vi "Handle.vi"(8 "error in (no error)":errorcluster, 11 "Instrument in":refnum<class "Instrument.lvclass">) -> (0 "error out":errorcluster, 3 "Instrument out":refnum<class "Instrument.lvclass">)   [LabVIEW 2018, in "Instrument.lvclass"]
uses:
  Instrument.lvclass
  C:/Users/devstaff/sparc4/s4gui/Versao ZeroMQ REQ-REP/SPARC4_GUI -v1.0.0 - 20250122_ICS-JSON/Server/Server.lvclass
  Server/Server.lvclass/Server.ctl
  Instrument.lvclass/Instrument.ctl
  Device/Device.lvclass/Device.ctl
  Device/Optics/Opt_Selector/Opt_Selector.lvclass
  C:/Users/devstaff/sparc4/s4gui/Versao ZeroMQ REQ-REP/SPARC4_GUI -v1.0.0 - 20250122_ICS-JSON/Device/Device.lvclass
  Device/Optics/Opt_Continuous/Opt_Continuous.lvclass
  Server/Server.lvclass
  Comm/Stream/Stream.lvclass
  Device/Device.lvclass
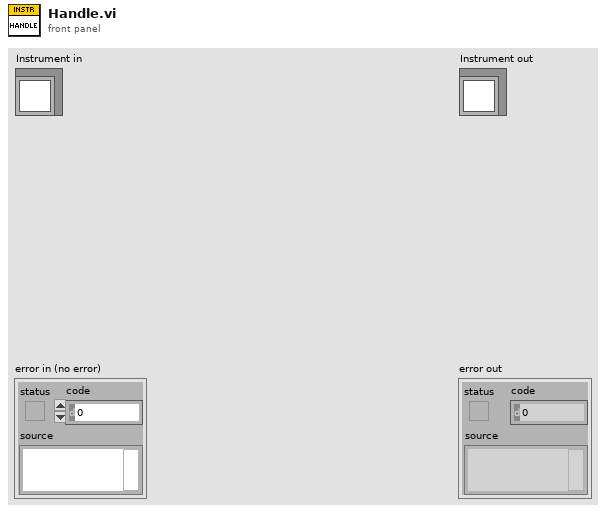
[diagram p1: front panel]
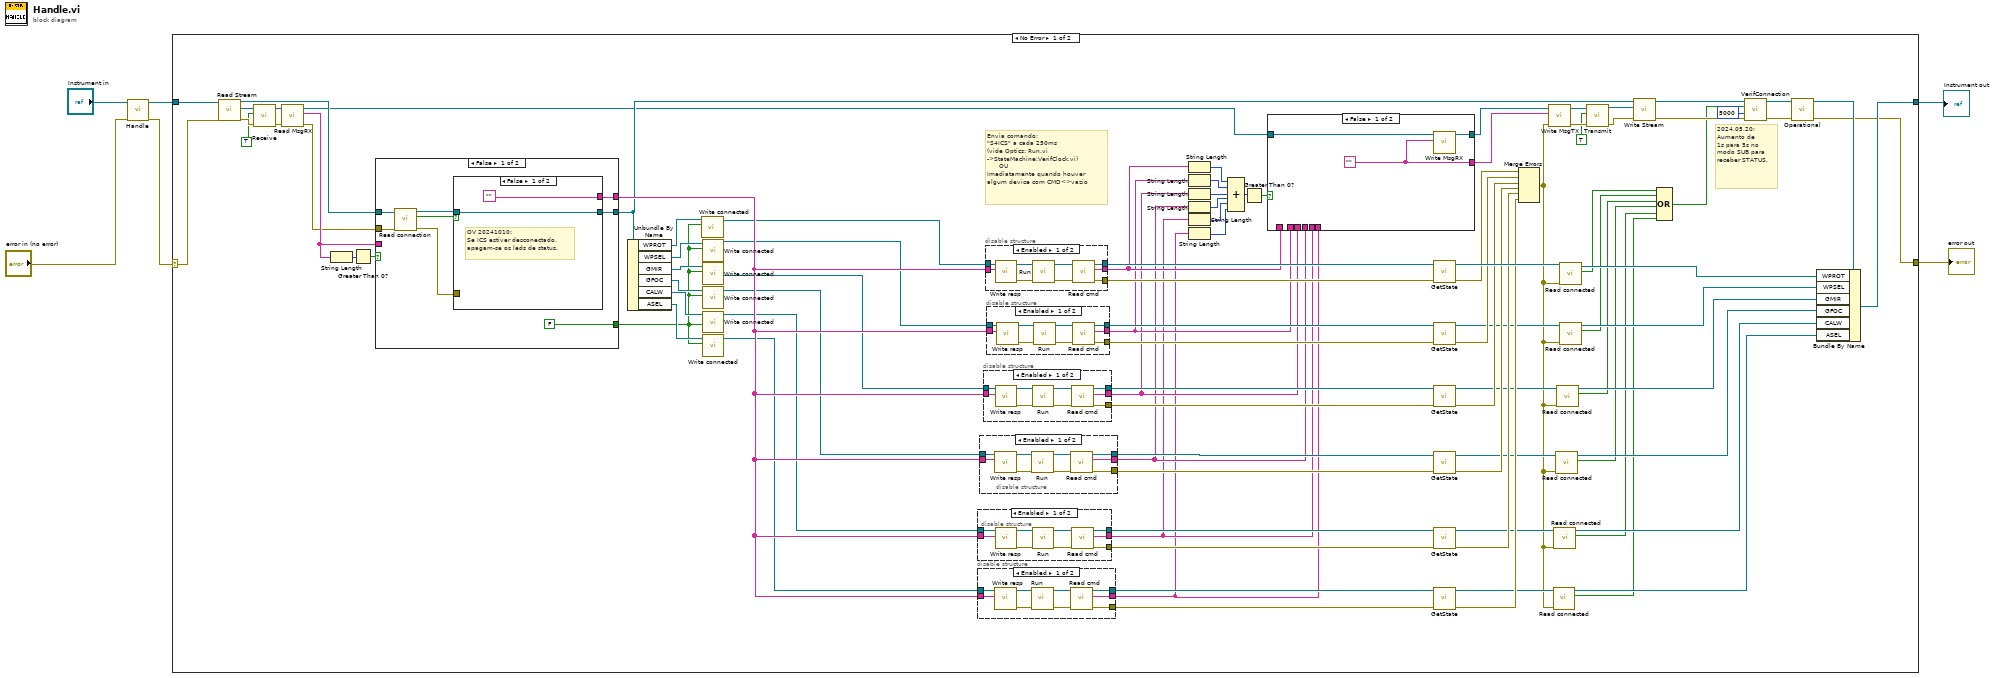
[diagram p0: block diagram]
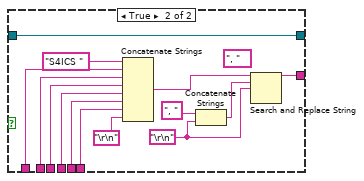
[diagram p2: hidden frame]
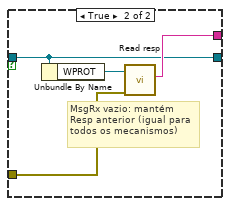
[diagram p3: hidden frame]
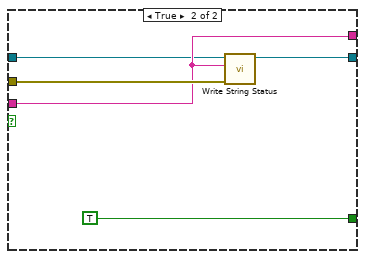
[diagram p4: hidden frame]
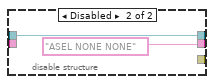
[diagram p5: hidden frame]
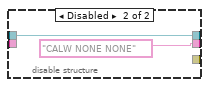
[diagram p6: hidden frame]
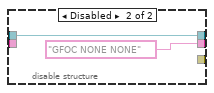
[diagram p7: hidden frame]
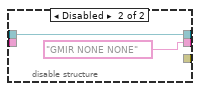
[diagram p8: hidden frame]
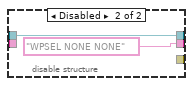
[diagram p9: hidden frame]
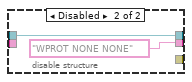
[diagram p10: hidden frame]
diagram:
  n1 = call-parent "Handle.vi"("error in (no error)"="error in (no error)", "Server in"="Instrument in") -> ("error out"=w3:errorcluster, "Server out"=w4:refnum<class "Instrument.lvclass">)  [unwired: 8 in]
  n2 = case shown="No Error" w3 {
    selector: w3 -> [w18 w205]
    tunnel: [w7 w205] -> w2
    tunnel: [w101 w204] -> w1
    tunnel: w4 -> [w17 w204]
    frame No Error {
      # "2024.05.20:\nAumento de \n1s para 5s no\nmodo SUB para\nreceber STATUS."
      # "Envia comando:\n\"S4ICS\" a cada 250ms\n(vide Optics: Run.vi\n->StateMachine:VerifClock.vi)\n      OU\nImediatamente quando houver\nalgum device com CMD<>vazio"
      n3 = call-dynamic "Read Stream.vi"("error in (no error)"=w18, "Server in"=w17) -> ("error out"=w99:errorcluster, "Stream.lvclass"=w100:refnum<class "Stream.lvclass">, "Server out"=w51:refnum<class "Instrument.lvclass">)  [unwired: 7 in]
      n4 = call-dynamic "Receive.vi"("error in (no error)"=w99, "log?"=TRUE, "Stream in"=w100) -> ("error out"=w98:errorcluster, "Stream out"=w97:refnum<class "Stream.lvclass">)  [unwired: 7 in]
      n5 = call-dynamic "Read MsgRX.vi"("error in (no error)"=w98, "Comm in"=w97) -> ("error out"=w49:errorcluster, "MsgRX"=w50:string, "Comm out"=w12:refnum<class "Stream.lvclass">)  [unwired: 7 in]
      n6 = String Length(string=w50) -> (length=w53:i32)
      n7 = Greater Than 0?(x=w53) -> (x > 0?=w52:bool)
      n8 = case shown="False" w52 {
        tunnel: [w119 w137] -> w39
        tunnel: w51 -> [w124 w134]
        tunnel: w50 -> [_ w135]
        tunnel: w49 -> [w123 w136]
        tunnel: [w126 w135] -> w47
        tunnel: [FALSE ("connected") TRUE ("connected")] -> w32
        frame False {
          n9 = call "Read connection.vi"("error in (no error)"=w123, "Server in"=w124) -> ("error out"=w122:errorcluster, "connection"=w120:bool, "Server out"=w121:refnum<class "Instrument.lvclass">)  [unwired: 7 in]
          n10 = case shown="False" w120 {
            tunnel: w121 -> [w127 w129]
            tunnel: ["" ("resp") w131] -> w126
            tunnel: w122 -> [_ w130]
            tunnel: [w127 w129] -> w119
            frame False {
              # "OV 20241010:\nSe ICS estiver desconectado, \napagam-se os leds de status."
            }
            frame True {
              # "MsgRx vazio: mantém \nResp anterior (igual para\ntodos os mecanismos)"
              n11 = Unbundle By Name(w129) -> ("WPROT"=w132:refnum<class "Opt_Selector.lvclass">)
              n12 = call-dynamic "Read resp.vi"("error in (no error)"=w130, "Device in"=w132) -> ("resp"=w131:string)  [unwired: 7 in, 2 out]
            }
          }
        }
        frame True {
          n13 = call-dynamic "Write String Status.vi"("error in (no error)"=w136, "String Status"=w135, "Server in"=w134) -> ("Server out"=w137:refnum<class "Instrument.lvclass">)  [unwired: 7 in, 1 out]
        }
      }
      n14 = Unbundle By Name(w39) -> ("WPROT"=w40:refnum<class "Opt_Selector.lvclass">, "WPSEL"=w41:refnum<class "Opt_Selector.lvclass">, "GMIR"=w42:refnum<class "Opt_Continuous.lvclass">, "GFOC"=w43:refnum<class "Opt_Continuous.lvclass">, "CALW"=w44:refnum<class "Opt_Selector.lvclass">, "ASEL"=w45:refnum<class "Opt_Selector.lvclass">)
      n15 = call "Write connected.vi"("connected"=w32, "Device in"=w40) -> ("Device out"=w38:refnum<class "Opt_Selector.lvclass">)  [unwired: 8 in, 1 out]
      n16 = call "Write connected.vi"("connected"=w32, "Device in"=w41) -> ("Device out"=w37:refnum<class "Opt_Selector.lvclass">)  [unwired: 8 in, 1 out]
      n17 = call "Write connected.vi"("connected"=w32, "Device in"=w42) -> ("Device out"=w36:refnum<class "Opt_Continuous.lvclass">)  [unwired: 8 in, 1 out]
      n18 = call "Write connected.vi"("connected"=w32, "Device in"=w43) -> ("Device out"=w35:refnum<class "Opt_Continuous.lvclass">)  [unwired: 8 in, 1 out]
      n19 = call "Write connected.vi"("connected"=w32, "Device in"=w44) -> ("Device out"=w34:refnum<class "Opt_Selector.lvclass">)  [unwired: 8 in, 1 out]
      n20 = call "Write connected.vi"("connected"=w32, "Device in"=w45) -> ("Device out"=w33:refnum<class "Opt_Selector.lvclass">)  [unwired: 8 in, 1 out]
      n21 = disable-structure shown="Enabled" {
        disable-tunnel: w34 -> [w157 w159]
        disable-tunnel: w47 -> [w156 _]
        disable-tunnel: [w155 "CALW NONE NONE" ("cmd")] -> w20
        disable-tunnel: [w154 w159] -> w78
        disable-tunnel: [w153 _] -> w77
        frame Enabled {
          n22 = call-dynamic "Write resp.vi"("resp"=w156, "Device in"=w157) -> ("error out"=w151:errorcluster, "Device out"=w152:refnum<class "Opt_Selector.lvclass">)  [unwired: 8 in]
          n23 = call-dynamic "Run.vi"("error in (no error)"=w151, "Opctics in"=w152) -> ("error out"=w150:errorcluster, "Opt_Selector out"=w149:refnum<class "Opt_Selector.lvclass">)  [unwired: 8 in]
          n24 = call-dynamic "Read cmd.vi"("error in (no error)"=w150, "Device in"=w149) -> ("error out"=w153:errorcluster, "cmd"=w155:string, "Device out"=w154:refnum<class "Opt_Selector.lvclass">)  [unwired: 7 in]
        }
        frame Disabled {
        }
      }
      n25 = disable-structure shown="Enabled" {
        disable-tunnel: w33 -> [w146 w148]
        disable-tunnel: w47 -> [w145 _]
        disable-tunnel: [w144 "ASEL NONE NONE" ("cmd")] -> w19
        disable-tunnel: [w143 w148] -> w75
        disable-tunnel: [w142 _] -> w74
        frame Enabled {
          n26 = call-dynamic "Write resp.vi"("resp"=w145, "Device in"=w146) -> ("error out"=w140:errorcluster, "Device out"=w141:refnum<class "Opt_Selector.lvclass">)  [unwired: 8 in]
          n27 = call-dynamic "Run.vi"("error in (no error)"=w140, "Opctics in"=w141) -> ("error out"=w139:errorcluster, "Opt_Selector out"=w138:refnum<class "Opt_Selector.lvclass">)  [unwired: 8 in]
          n28 = call-dynamic "Read cmd.vi"("error in (no error)"=w139, "Device in"=w138) -> ("error out"=w142:errorcluster, "cmd"=w144:string, "Device out"=w143:refnum<class "Opt_Selector.lvclass">)  [unwired: 7 in]
        }
        frame Disabled {
        }
      }
      n29 = disable-structure shown="Enabled" {
        disable-tunnel: w35 -> [w168 w170]
        disable-tunnel: w47 -> [w167 _]
        disable-tunnel: [w166 "GFOC NONE NONE" ("cmd")] -> w21
        disable-tunnel: [w165 w170] -> w81
        disable-tunnel: [w164 _] -> w80
        frame Enabled {
          n30 = call-dynamic "Write resp.vi"("resp"=w167, "Device in"=w168) -> ("error out"=w162:errorcluster, "Device out"=w163:refnum<class "Opt_Continuous.lvclass">)  [unwired: 8 in]
          n31 = call-dynamic "Run.vi"("error in (no error)"=w162, "Opctics in"=w163) -> ("error out"=w161:errorcluster, "Opt_Continuous out"=w160:refnum<class "Opt_Continuous.lvclass">)  [unwired: 8 in]
          n32 = call-dynamic "Read cmd.vi"("error in (no error)"=w161, "Device in"=w160) -> ("error out"=w164:errorcluster, "cmd"=w166:string, "Device out"=w165:refnum<class "Opt_Continuous.lvclass">)  [unwired: 7 in]
        }
        frame Disabled {
        }
      }
      n33 = disable-structure shown="Enabled" {
        disable-tunnel: w36 -> [w179 w181]
        disable-tunnel: w47 -> [w178 _]
        disable-tunnel: [w177 "GMIR NONE NONE" ("cmd")] -> w22
        disable-tunnel: [w176 w181] -> w84
        disable-tunnel: [w175 _] -> w83
        frame Enabled {
          n34 = call-dynamic "Write resp.vi"("resp"=w178, "Device in"=w179) -> ("error out"=w173:errorcluster, "Device out"=w174:refnum<class "Opt_Continuous.lvclass">)  [unwired: 8 in]
          n35 = call-dynamic "Run.vi"("error in (no error)"=w173, "Opctics in"=w174) -> ("error out"=w172:errorcluster, "Opt_Continuous out"=w171:refnum<class "Opt_Continuous.lvclass">)  [unwired: 8 in]
          n36 = call-dynamic "Read cmd.vi"("error in (no error)"=w172, "Device in"=w171) -> ("error out"=w175:errorcluster, "cmd"=w177:string, "Device out"=w176:refnum<class "Opt_Continuous.lvclass">)  [unwired: 7 in]
        }
        frame Disabled {
        }
      }
      n37 = disable-structure shown="Enabled" {
        disable-tunnel: w38 -> [w201 w203]
        disable-tunnel: [w200 _] -> w90
        disable-tunnel: w47 -> [w199 _]
        disable-tunnel: [w198 "WPROT NONE NONE" ("cmd")] -> w24
        disable-tunnel: [w197 w203] -> w46
        frame Enabled {
          n38 = call-dynamic "Write resp.vi"("resp"=w199, "Device in"=w201) -> ("error out"=w195:errorcluster, "Device out"=w196:refnum<class "Opt_Selector.lvclass">)  [unwired: 8 in]
          n39 = call-dynamic "Run.vi"("error in (no error)"=w195, "Opctics in"=w196) -> ("error out"=w194:errorcluster, "Opt_Selector out"=w193:refnum<class "Opt_Selector.lvclass">)  [unwired: 8 in]
          n40 = call-dynamic "Read cmd.vi"("error in (no error)"=w194, "Device in"=w193) -> ("error out"=w200:errorcluster, "cmd"=w198:string, "Device out"=w197:refnum<class "Opt_Selector.lvclass">)  [unwired: 7 in]
        }
        frame Disabled {
        }
      }
      n41 = disable-structure shown="Enabled" {
        disable-tunnel: w37 -> [w190 w192]
        disable-tunnel: [w189 w192] -> w87
        disable-tunnel: [w188 _] -> w86
        disable-tunnel: w47 -> [w187 _]
        disable-tunnel: [w186 "WPSEL NONE NONE" ("cmd")] -> w23
        frame Enabled {
          n42 = call-dynamic "Write resp.vi"("resp"=w187, "Device in"=w190) -> ("error out"=w184:errorcluster, "Device out"=w185:refnum<class "Opt_Selector.lvclass">)  [unwired: 8 in]
          n43 = call-dynamic "Run.vi"("error in (no error)"=w184, "Opctics in"=w185) -> ("error out"=w183:errorcluster, "Opt_Selector out"=w182:refnum<class "Opt_Selector.lvclass">)  [unwired: 8 in]
          n44 = call-dynamic "Read cmd.vi"("error in (no error)"=w183, "Device in"=w182) -> ("error out"=w188:errorcluster, "cmd"=w186:string, "Device out"=w189:refnum<class "Opt_Selector.lvclass">)  [unwired: 7 in]
        }
        frame Disabled {
        }
      }
      n45 = String Length(string=w24) -> (length=w31:i32)
      n46 = String Length(string=w23) -> (length=w30:i32)
      n47 = String Length(string=w22) -> (length=w29:i32)
      n48 = String Length(string=w21) -> (length=w28:i32)
      n49 = String Length(string=w20) -> (length=w27:i32)
      n50 = String Length(string=w19) -> (length=w26:i32)
      n51 = Compound Arithmetic op=ADD(w31, w30, w29, w28, w27, w26) -> (w25:i32)
      n52 = Greater Than 0?(x=w25) -> (x > 0?=w13:bool)
      n53 = case shown="False" w13 {
        tunnel: w24 -> [_ w118]
        tunnel: w23 -> [_ w117]
        tunnel: w22 -> [_ w116]
        tunnel: w21 -> [_ w115]
        tunnel: w20 -> [_ w114]
        tunnel: w19 -> [_ w111]
        tunnel: [w103 w106] -> w48
        tunnel: w12 -> [w104 w105]
        tunnel: [w102 w105] -> w11
        frame False {
          w103 = "" ("result string")
          n54 = call-dynamic "Write MsgRX.vi"("MsgRX"=w103, "Comm in"=w104) -> ("Comm out"=w102:refnum<class "Stream.lvclass">)  [unwired: 8 in, 1 out]
        }
        frame True {
          w107 = "\r\n"
          (unwired) ", " ("string")
          n55 = Concatenate Strings("S4ICS " ("string"), w118, w117, w116, w115, w114, w111, "\r\n") -> (w108:string)
          n56 = Concatenate Strings(", " ("search string"), w107) -> (w109:string)
          n57 = Search and Replace String(input string=w108, search string=w109, replace string=w107) -> (result string=w106:string)  [unwired: 5 in, 3 out]
        }
      }
      n58 = call-dynamic "GetState.vi"("error in (no error)"=w90, "Optics in"=w46) -> ("error out"=w88:errorcluster, "Optics out"=w89:refnum<class "Opt_Selector.lvclass">)  [unwired: 8 in]
      n59 = call-dynamic "GetState.vi"("error in (no error)"=w86, "Optics in"=w87) -> ("error out"=w85:errorcluster, "Optics out"=w72:refnum<class "Opt_Selector.lvclass">)  [unwired: 8 in]
      n60 = call-dynamic "GetState.vi"("error in (no error)"=w83, "Optics in"=w84) -> ("error out"=w82:errorcluster, "Optics out"=w68:refnum<class "Opt_Continuous.lvclass">)  [unwired: 8 in]
      n61 = call-dynamic "GetState.vi"("error in (no error)"=w80, "Optics in"=w81) -> ("error out"=w79:errorcluster, "Optics out"=w66:refnum<class "Opt_Continuous.lvclass">)  [unwired: 8 in]
      n62 = call-dynamic "GetState.vi"("error in (no error)"=w77, "Optics in"=w78) -> ("error out"=w76:errorcluster, "Optics out"=w62:refnum<class "Opt_Selector.lvclass">)  [unwired: 8 in]
      n63 = call-dynamic "GetState.vi"("error in (no error)"=w74, "Optics in"=w75) -> ("error out"=w73:errorcluster, "Optics out"=w60:refnum<class "Opt_Selector.lvclass">)  [unwired: 8 in]
      n64 = Merge Errors(w88, w85, w82, w79, w76, w73) -> (w56:errorcluster)
      n65 = call-dynamic "Write MsgTX.vi"("error in (no error)"=w56, "MsgTX"=w48, "Comm in"=w11) -> ("error out"=w95:errorcluster, "Comm out"=w96:refnum<class "Stream.lvclass">)  [unwired: 7 in]
      n66 = call "Read connected.vi"("error in (no error)"=w56, "Device in"=w60) -> ("connected"=w57:bool, "Device out"=w59:refnum<class "Opt_Selector.lvclass">)  [unwired: 7 in, 1 out]
      n67 = call "Read connected.vi"("error in (no error)"=w56, "Device in"=w62) -> ("connected"=w58:bool, "Device out"=w61:refnum<class "Opt_Selector.lvclass">)  [unwired: 7 in, 1 out]
      n68 = call "Read connected.vi"("error in (no error)"=w56, "Device in"=w66) -> ("connected"=w63:bool, "Device out"=w65:refnum<class "Opt_Continuous.lvclass">)  [unwired: 7 in, 1 out]
      n69 = call "Read connected.vi"("error in (no error)"=w56, "Device in"=w68) -> ("connected"=w64:bool, "Device out"=w67:refnum<class "Opt_Continuous.lvclass">)  [unwired: 7 in, 1 out]
      n70 = call "Read connected.vi"("error in (no error)"=w56, "Device in"=w89) -> ("connected"=w70:bool, "Device out"=w92:refnum<class "Opt_Selector.lvclass">)  [unwired: 7 in, 1 out]
      n71 = call "Read connected.vi"("error in (no error)"=w56, "Device in"=w72) -> ("connected"=w69:bool, "Device out"=w71:refnum<class "Opt_Selector.lvclass">)  [unwired: 7 in, 1 out]
      n72 = call-dynamic "Transmit.vi"("error in (no error)"=w95, "log?"=TRUE, "Stream in"=w96) -> ("error out"=w93:errorcluster, "Stream out"=w94:refnum<class "Stream.lvclass">)  [unwired: 7 in]
      n73 = call-dynamic "Write Stream.vi"("error in (no error)"=w93, "Stream.lvclass"=w94, "Server in"=w39) -> ("error out"=w91:errorcluster, "Server out"=w54:refnum<class "Instrument.lvclass">)  [unwired: 7 in]
      n74 = Compound Arithmetic op=OR(w70, w69, w64, w63, w58, w57) -> (w55:bool)
      n75 = call-dynamic "VerifConnection.vi"("error in (no error)"=w91, "timeout in ms (1000)"=u32 5000, "device connected in"=w55, "Server in"=w54) -> ("error out"=w9:errorcluster, "Server out"=w10:refnum<class "Instrument.lvclass">)  [unwired: 6 in]
      n76 = call-dynamic "Operational.vi"("error in (no error)"=w9, "Instrument in"=w10) -> ("error out"=w7:errorcluster, "Instrument out"=w8:refnum<class "Instrument.lvclass">)  [unwired: 8 in]
      n77 = Bundle By Name(cluster=w8, "WPROT"=w92, "WPSEL"=w71, "GMIR"=w67, "GFOC"=w65, "CALW"=w61, "ASEL"=w59) -> (w101:refnum<class "Instrument.lvclass">)
    }
    frame Error {
    }
  }
  "error out" <- w2
  "Instrument out" <- w1
